vi "Readings Test (FPGA).vi"() -> ()   [LabVIEW 2013]
uses:
  <vilib>/rvi/Emulation/niFpgaSctlEmulationGetInTimedLoop.vi
  <vilib>/rvi/Emulation/niFpgaEmulationReportErrorSimple.vi
  <vilib>/rvi/Emulation/niFpgaGetClockAttributes.vi
  <vilib>/rvi/Emulation/niFpgaCriticalErrorInLSC.vi
  <vilib>/rvi/DataTransferAndStorage/Container/Common/niFpgaContainerExecOnDevCompGetState.vi
  <vilib>/rvi/FIFO/Fifo_Resource/nirvififoEmulationWriteFpgaImpl.vi
  <vilib>/rvi/DataTransferAndStorage/Container/Common/niFpgaContainerGetUniqueNameForEmu.vi
  <vilib>/rvi/interface/RandomDataEmulation/nirviRandomDataFPGAFIFO.vi
  <vilib>/rvi/interface/RandomDataEmulation/niFpgaRandomDataHandleErrors.vi
  <vilib>/rvi/eio/common/nirviEmuReportErrorAndStop.vi
  <vilib>/rvi/DataTransferAndStorage/Container/XNode/niFpgaContainer.xnode
  <vilib>/rvi/FIFO/Fifo_Resource/niFpgaFifoEmulationRefIn.vi
  <vilib>/eio/EIONode/EIONode.xnode
  <vilib>/rvi/eio/common/nirviEmuTemplateMethod_errors.vi
panel:
  out "ticks/loop 2":u32
  out "sine out 6":i16
  out "sine out 5":i16
  out "sine out 4":i16
  out "sine out 3":i16
  out "sine out 2":i16
  out "sine out":i16
  out "ticks/loop 1":u32
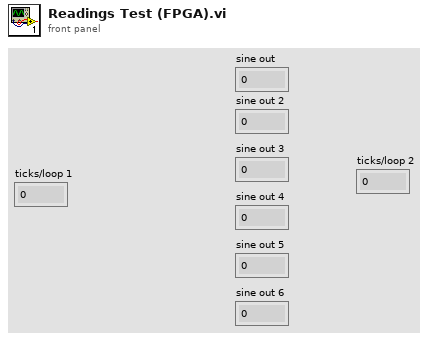
[diagram p1: front panel]
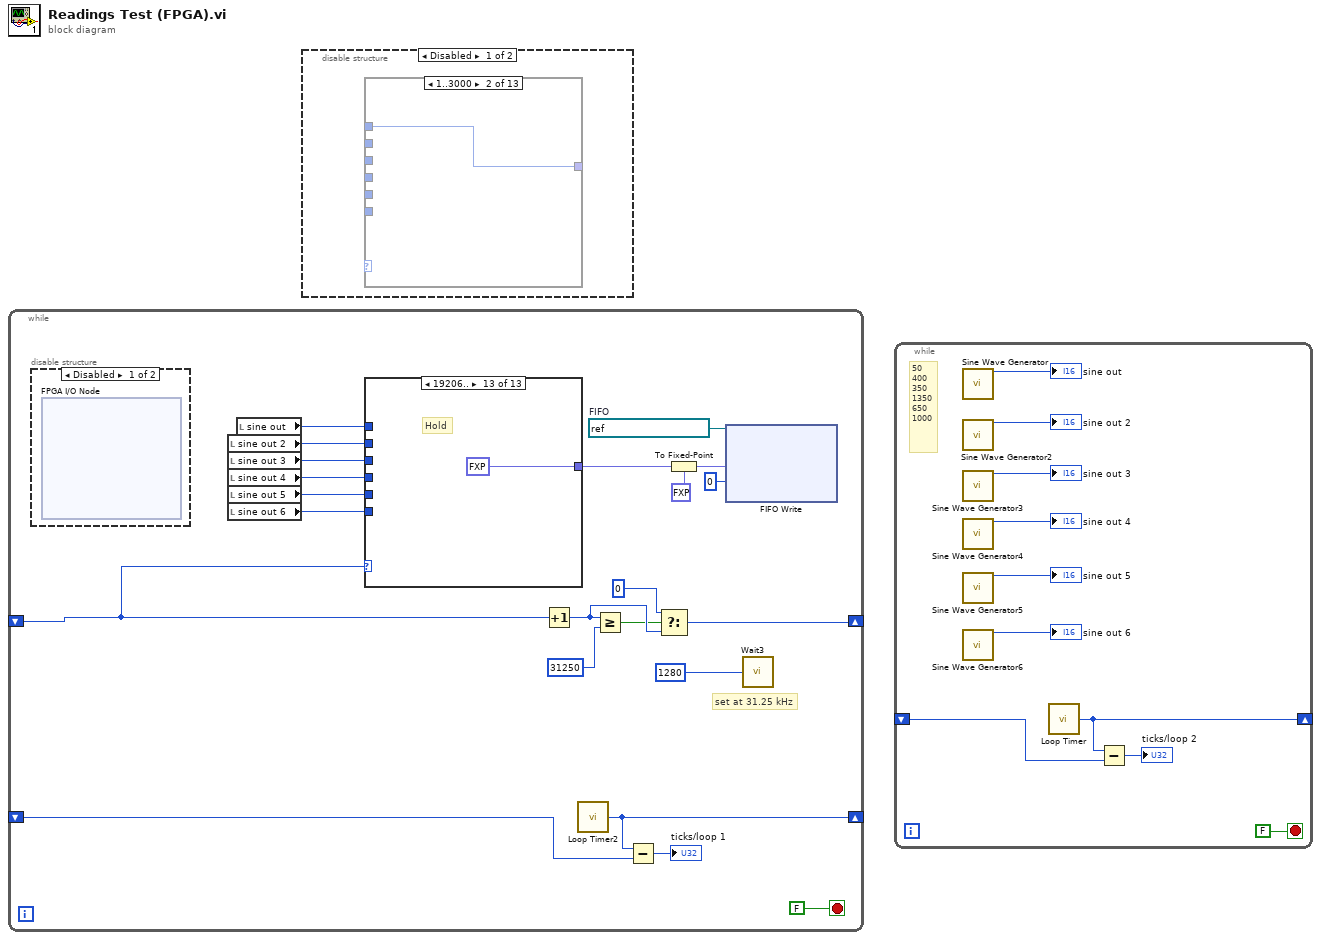
[diagram p0: block diagram]
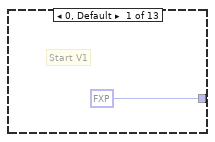
[diagram p2: hidden frame]
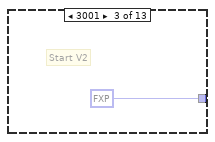
[diagram p3: hidden frame]
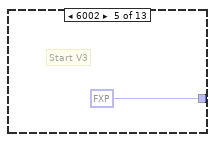
[diagram p5: hidden frame]
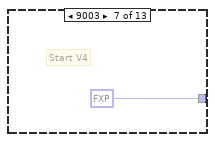
[diagram p7: hidden frame]
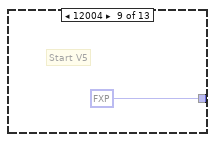
[diagram p9: hidden frame]
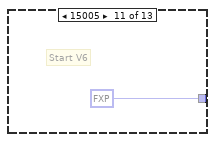
[diagram p11: hidden frame]
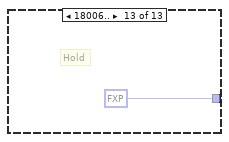
[diagram p13: hidden frame]
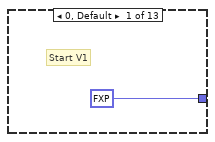
[diagram p16: hidden frame]
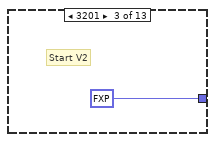
[diagram p18: hidden frame]
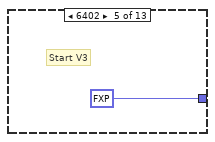
[diagram p20: hidden frame]
diagram:
  n1 = while {
    shift-right: [w22] -> _
    shift-left: _ -> [w21]
    shift-right: [w11] -> _
    shift-left: _ -> [w10]
    stop <- FALSE stop-if-true
    w18 = refnum<k21> "Voltage for Speed"  # FIFO
    # "set at 31.25 kHz"
    n2 = disable-structure shown="Disabled" {
      frame Disabled {
        n3 = xnode "FPGA I/O Node"() -> ()  [unwired: 6 in, 12 out]
      }
      frame Enabled {
      }
    }
    n4 = local read "sine out 2"() -> (w5:i16)
    n5 = local read "sine out 3"() -> (w4:i16)
    n6 = local read "sine out 4"() -> (w3:i16)
    n7 = local read "sine out 5"() -> (w2:i16)
    n8 = local read "sine out 6"() -> (w1:i16)
    n9 = local read "sine out"() -> (w6:i16)
    n10 = case shown="19206.." w21 {
      tunnel: [fxp<+/-,25,6> -21.0 ("Controller_Current_1 (AI6)") w24 fxp<+/-,25,6> -22.0 ("Controller_Current_1 (AI6)") w26 fxp<+/-,25,6> -23.0 ("Controller_Current_1 (AI6)") w28 fxp<+/-,25,6> -24.0 ("Controller_Current_1 (AI6)") w30 fxp<+/-,25,6> -25.0 ("Controller_Current_1 (AI6)") w32 fxp<+/-,25,6> -26.0 ("Controller_Current_1 (AI6)") w34 fxp<+/-,25,6> -31.0 ("Controller_Current_1 (AI6)")] -> w16
      tunnel: w6 -> [_ w24 _ _ _ _ _ _ _ _ _ _ _]
      tunnel: w5 -> [_ _ _ w26 _ _ _ _ _ _ _ _ _]
      tunnel: w4 -> [_ _ _ _ _ w28 _ _ _ _ _ _ _]
      tunnel: w3 -> [_ _ _ _ _ _ _ w30 _ _ _ _ _]
      tunnel: w2 -> [_ _ _ _ _ _ _ _ _ w32 _ _ _]
      tunnel: w1 -> [_ _ _ _ _ _ _ _ _ _ _ w34 _]
      frame 0, Default {
        # "Start V1"
      }
      frame 1..3200 {
      }
      frame 3201 {
        # "Start V2"
      }
      frame 3202..6401 {
      }
      frame 6402 {
        # "Start V3"
      }
      frame 6403..9602 {
      }
      frame 9603 {
        # "Start V4"
      }
      frame 9604..12803 {
      }
      frame 12804 {
        # "Start V5"
      }
      frame 12805..16004 {
      }
      frame 16005 {
        # "Start V6"
      }
      frame 16006..19205 {
      }
      frame 19206.. {
        # "Hold"
      }
    }
    n11 = Increment(x=w21) -> (x+1=w15:i32)
    n12 = call "Loop Timer2"() -> ("Tick Count(Ticks)"=w11:u32)  [unwired: 1 in]
    n13 = Greater Or Equal?(x=w15, y=31250) -> (x >= y?=w13:bool)
    n14 = Subtract(x=w11, y=w10) -> (x-y=→"ticks/loop 1":u32)
    n15 = Select(t=0, s=w13, f=w15) -> (s? t:f=w22:i32)
    n16 = To Fixed-Point(fixed-point type=fxp<+/-,25,6> 0.0 ("Controller_Current_1 (AI6)"), number=w16) -> (fixed-point=w19:fxp<+/-,25,6>)
    n17 = xnode ("FIFO Write")("Element"=w19, "Timeout"=0, "FIFO In"=w18) -> ()  [unwired: 2 out]
    n18 = call "Wait3"("Count(Ticks)"=u32 1280 ("Count(mSec)")) -> ()  [unwired: 1 out]
  }
  n19 = disable-structure shown="Disabled" {
    frame Disabled {
      n20 = case shown="1..3000" {
        selector: _ -> [_ _ _ _ _ _ _ _ _ _ _ _ _]
        tunnel: [fxp<+/-,25,6> -21.0 ("Controller_Current_1 (AI6)") w37 fxp<+/-,25,6> -22.0 ("Controller_Current_1 (AI6)") w39 fxp<+/-,25,6> -23.0 ("Controller_Current_1 (AI6)") w41 fxp<+/-,25,6> -24.0 ("Controller_Current_1 (AI6)") w43 fxp<+/-,25,6> -25.0 ("Controller_Current_1 (AI6)") w45 fxp<+/-,25,6> -26.0 ("Controller_Current_1 (AI6)") w47 fxp<+/-,25,6> -31.0 ("Controller_Current_1 (AI6)")] -> _
        tunnel: _ -> [_ w37 _ _ _ _ _ _ _ _ _ _ _]
        tunnel: _ -> [_ _ _ w39 _ _ _ _ _ _ _ _ _]
        tunnel: _ -> [_ _ _ _ _ w41 _ _ _ _ _ _ _]
        tunnel: _ -> [_ _ _ _ _ _ _ w43 _ _ _ _ _]
        tunnel: _ -> [_ _ _ _ _ _ _ _ _ w45 _ _ _]
        tunnel: _ -> [_ _ _ _ _ _ _ _ _ _ _ w47 _]
        frame 0, Default {
          # "Start V1"
        }
        frame 1..3000 {
        }
        frame 3001 {
          # "Start V2"
        }
        frame 3002..6001 {
        }
        frame 6002 {
          # "Start V3"
        }
        frame 6003..9002 {
        }
        frame 9003 {
          # "Start V4"
        }
        frame 9004..12003 {
        }
        frame 12004 {
          # "Start V5"
        }
        frame 12005..15004 {
        }
        frame 15005 {
          # "Start V6"
        }
        frame 15006..18005 {
        }
        frame 18006.. {
          # "Hold"
        }
      }
    }
    frame Enabled {
    }
  }
  n21 = while {
    shift-right: [w50] -> _
    shift-left: _ -> [w49]
    stop <- FALSE stop-if-true
    # "50\n400\n350\n1350\n650\n1000"
    n22 = call "Sine Wave Generator"() -> ("sine out"=→"sine out":i16)  [unwired: 15 in]
    n23 = call "Sine Wave Generator2"() -> ("sine out"=→"sine out 2":i16)  [unwired: 15 in]
    n24 = call "Sine Wave Generator3"() -> ("sine out"=→"sine out 3":i16)  [unwired: 15 in]
    n25 = call "Sine Wave Generator4"() -> ("sine out"=→"sine out 4":i16)  [unwired: 15 in]
    n26 = call "Sine Wave Generator5"() -> ("sine out"=→"sine out 5":i16)  [unwired: 15 in]
    n27 = call "Sine Wave Generator6"() -> ("sine out"=→"sine out 6":i16)  [unwired: 15 in]
    n28 = call "Loop Timer"() -> ("Tick Count(Ticks)"=w50:u32)  [unwired: 1 in]
    n29 = Subtract(x=w50, y=w49) -> (x-y=→"ticks/loop 2":u32)
  }
